vi "Update Clone ID in Tree.vi"(6 "Clone ID":string, 8 "error in (no error)":errorcluster, 9 "DC_UID":T1, 10 "WID":string, 11 "Tree Ref":refnum<vi>) -> (0 "error out":errorcluster)   [LabVIEW 2017, in "Application Manager.lvclass"]
uses:
  Application Manager.lvclass
  Common VIs/DC_UID.ctl
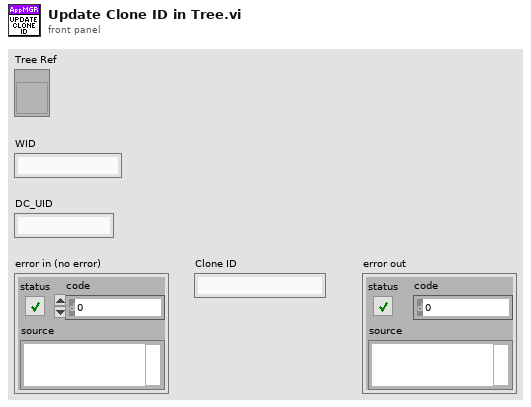
[diagram p1: front panel]
types:
  T1 = typedef "DC_UID.ctl" = string
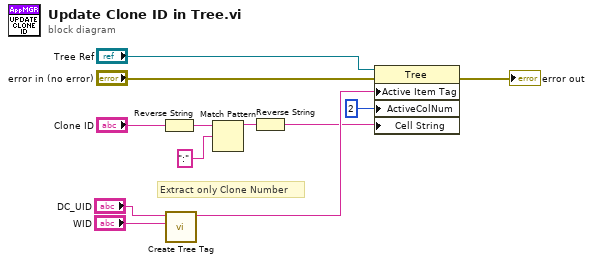
[diagram p0: block diagram]
diagram:
  # "Extract only Clone Number"
  n1 = Reverse String(1:"Clone ID") -> (0:w3:string)
  n2 = call "Create Tree Tag.vi"("WID"="WID", "DC_UID"="DC_UID") -> ("Tree Tag"=w6:string)  [unwired: 9 in]
  n3 = Match Pattern(string=w3, regular expression=":") -> (before substring=w5:string)  [unwired: 1 in, 3 out]
  n4 = Reverse String(1:w5) -> (0:w1:string)
  n5 = property class="Tree"(reference="Tree Ref", error in="error in (no error)", "Active Item Tag"=w6, "ActiveColNum"=2 ("Active Cell:Active Column Number"), "Cell String"=w1) -> (error out=→"error out":errorcluster)  [unwired: 1 out]
